vi "RESTful OutputType To Text.vi"(1 "Output format":T1) -> (0 "Boolean Text":string)   [LabVIEW 2020]
uses:
  <vilib>/AppBuilder/AB_Classes/Source/RESTfulVI/Configure_RESTfulVI/AB_RESTful_OutputFormat.ctl
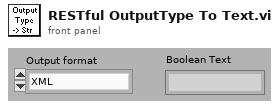
[diagram p1: front panel]
types:
  T1 = typedef "AB_RESTful_OutputFormat.ctl" = enum32{"XML", "Text", "HTML", "JSON"}
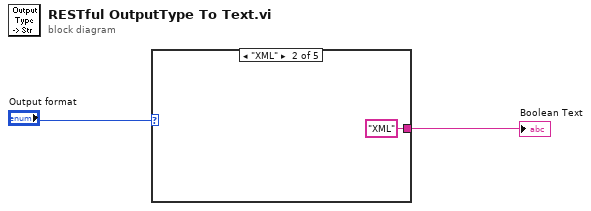
[diagram p0: block diagram]
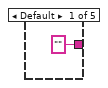
[diagram p2: hidden frame]
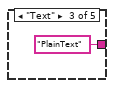
[diagram p3: hidden frame]
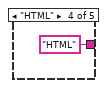
[diagram p4: hidden frame]
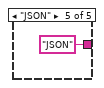
[diagram p5: hidden frame]
diagram:
  n1 = case shown="\"XML\"" "Output format" {
    tunnel: ["" ("Boolean Text") "XML" ("Boolean Text") "PlainText" ("Boolean Text") "HTML" ("Boolean Text") "JSON" ("Boolean Text")] -> w2
    frame Default {
    }
    frame "XML" {
    }
    frame "Text" {
    }
    frame "HTML" {
    }
    frame "JSON" {
    }
  }
  "Boolean Text" <- w2
